vi "Digitizer Output.vi"(10 "Digitizer 2":dbl[](array[numeric]), 11 "Digitizer 1":dbl[](array[numeric])) -> (3 "Digitizer Output":dbl[](array[numeric]))   [LabVIEW 2010]
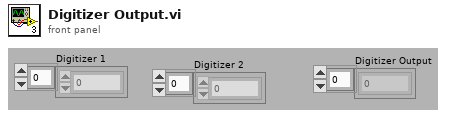
[diagram p1: front panel]
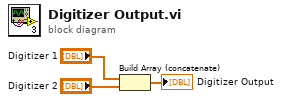
[diagram p0: block diagram]
diagram:
  n1 = Build Array (concatenate)("Digitizer 1", "Digitizer 2") -> (→"Digitizer Output":dbl[])
